vi "Image Process ConvertingToUDP.vi"(0 "Particle Measurements (Pixels)":dbl[][](array[numeric])) -> (7 "String":string)   [LabVIEW 2012]
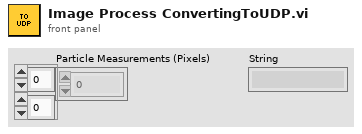
[diagram p1: front panel]
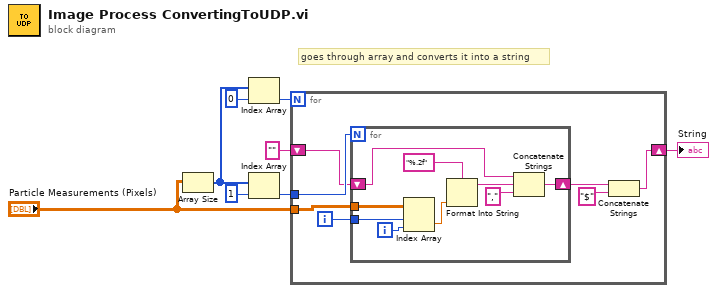
[diagram p0: block diagram]
diagram:
  # "goes through array and converts it into a string"
  n1 = Array Size(array="Particle Measurements (Pixels)") -> (size(s)=w5:i32[])
  n2 = Index Array(array=w5, index=0) -> (element=w3:i32)
  n3 = Index Array(array=w5, index=1) -> (element=w6:i32)
  n4 = for {
    N: w3 -> [_]
    tunnel: w6 -> [w15]
    shift-right: [w9] -> w8
    shift-left: "" -> [w14]
    tunnel: "Particle Measurements (Pixels)" -> [w13]
    i -> [w12]
    n5 = for {
      N: w15 -> [_]
      shift-right: [w23] -> w11
      shift-left: w14 -> [w24]
      tunnel: w13 -> [w21]
      tunnel: w12 -> [w20]
      i -> [w19]
      n6 = Index Array(array=w21, index (row)=w20, index (col)=w19) -> (element=w18:dbl)
      n7 = Format Into String(format string="%.2f", w18) -> (resulting string=w17:string)  [unwired: 2 in, 1 out]
      n8 = Concatenate Strings(w24, w17, "," ("string")) -> (w23:string)
    }
    n9 = Concatenate Strings(w11, "$" ("string")) -> (w9:string)
  }
  "String" <- w8
